vi "DriveAngleH.vi"(2 "Parameter String":string, 3 "Reinit":bool) -> (0 "Error Out":errorcluster, 1 "Increment":bool)   [LabVIEW 2020]
doc: "The swerve drive base will rotate about its center at a speed specified by the joystick command. This is a \"dumb\" algorithm, there is no feedback controller and the direction of rotation must be specified manually. Any complex or critical turns should be handled using either the Path Follower or auto-targeting. \n\nParameters:\n1. field-centric angle --> (deg) [0,360]\n2. relative rotation speed --> [-1,1]"
uses:
  SafeParser_Float.vi
  drivercommands.vi
  sensordata.vi
  autonomousinfo.vi
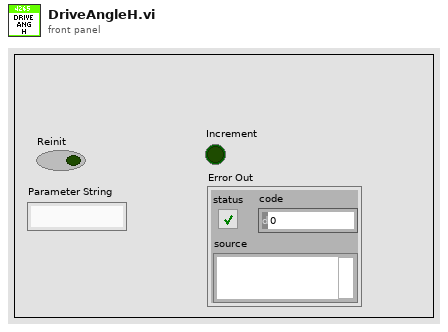
[diagram p1: front panel]
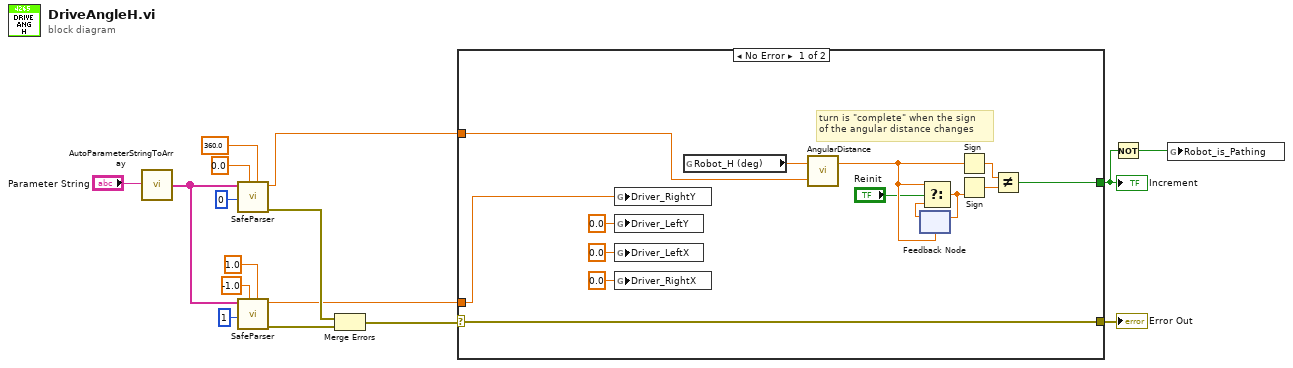
[diagram p0: block diagram]
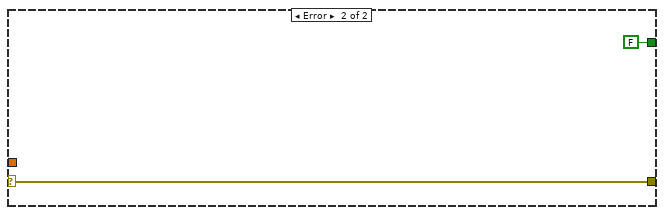
[diagram p2: hidden frame]
diagram:
  n1 = call "AutoParameterStringToArray.vi"("Parameter String"="Parameter String") -> ("Parsed Parameters"=w10:string[])
  n2 = call-poly "SafeParser.vi"("Maximum"=360.0, "Minimum"=0.0, "Array Index"=0 ("Parameter Index"), "String Array"=w10) -> ("Error Out"=w8:errorcluster, "Typecast  Value"=w6:dbl)  [unwired: 6 in]
  n3 = call-poly "SafeParser.vi"("Maximum"=1.0, "Minimum"=-1.0, "Array Index"=1 ("Parameter Index"), "String Array"=w10) -> ("Error Out"=w7:errorcluster, "Typecast  Value"=w5:dbl)  [unwired: 6 in]
  n4 = Merge Errors(w8, w7) -> (w9:errorcluster)
  n5 = case shown="No Error" w9 {
    selector: w9 -> [w21 w32]
    tunnel: [w17 FALSE] -> w1
    tunnel: [w21 w32] -> w16
    tunnel: w6 -> [w19 _]
    tunnel: w5 -> [w20 _]
    frame No Error {
      # "turn is \"complete\" when the sign\nof the angular distance changes"
      n6 = global write "drivercommands.vi" "Driver_RightY"(w20) -> ()
      n7 = global write "drivercommands.vi" "Driver_LeftY"(0.0 ("Driver_RightX")) -> ()
      n8 = global write "drivercommands.vi" "Driver_LeftX"(0.0 ("Driver_RightX")) -> ()
      n9 = global write "drivercommands.vi" "Driver_RightX"(0.0 ("Driver_RightX")) -> ()
      n10 = global read "sensordata.vi" "Robot_H (deg)"() -> (w18:dbl)
      n11 = call "AngularDistance.vi"("Goal Angle (deg) [0,360]"=w19, "Current Angle (deg) [-Inf,+Inf]"=w18) -> ("Signed Angular Distance (deg) [-180,+180]"=w25:dbl)  [unwired: 1 out]
      n12 = feedback #1(w25) -> (w26:dbl)
      n13 = Select(t=w25, s="Reinit", f=w26) -> (s? t:f=w27:dbl)
      n14 = feedback-in #1(w27) -> ()
      n15 = Sign(1:w25) -> (0:w23:dbl)
      n16 = Sign(1:w27) -> (0:w24:dbl)
      n17 = Not Equal?(x=w23, y=w24) -> (x != y?=w17:bool)
    }
    frame Error {
    }
  }
  "Increment" <- w1
  "Error Out" <- w16
  n18 = Not(x=w1) -> (.not. x?=w2:bool)
  n19 = global write "autonomousinfo.vi" "Robot_is_Pathing"(w2) -> ()
